vi "VI SysLoad.vi"() -> ()   [LabVIEW 2020, in "Erweiterte Konfig.lvlib" / "System Load.lvlib"]
uses:
  System Load.lvlib
  CPU Status.ctl
  CPU Speicher Auslastung.ctl
  <vilib>/nisyscfg/Close (System).vi
  Allgemein/allgemeine Sub-VIs.lvlib
  <vilib>/nisyscfg/nisyscfg.lvlib
  cRIO/PC/Kommunikation mit cRIO.lvlib
panel:
  out "CPU 2 Load:":T1
  out "Speicher":T2 caption="Memory:"
  out "CPU 1 Load":T1 caption="CPU 1 Load:"
  # "System Load"
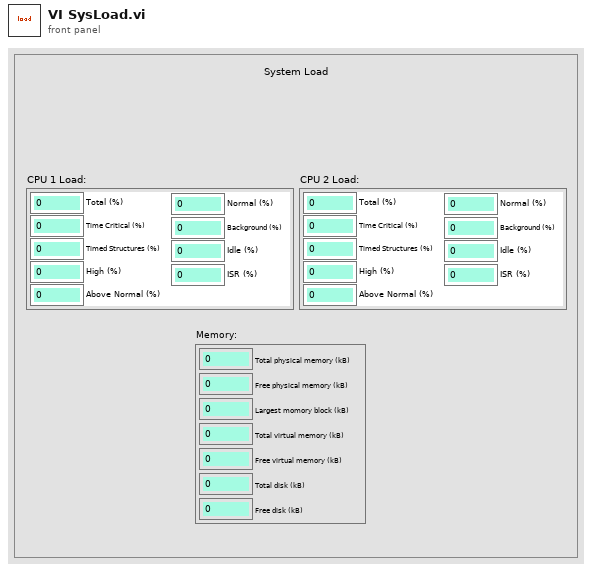
[diagram p1: front panel]
types:
  T1 = typedef "Erweiterte Konfig.lvlib/System Load.lvlib/CPU Status.ctl" = cluster{"Total (%)":sgl, "Time Critical (%)":sgl, "Timed Structures (%)":sgl, "High (%)":sgl, "Above Normal (%)":sgl, "Normal (%)":sgl, "Background (%)":sgl, "Idle (%)":sgl, "ISR (%)":sgl}
  T2 = typedef "Erweiterte Konfig.lvlib/System Load.lvlib/CPU Speicher Auslastung.ctl" = cluster{"Total physical memory (kB)":u32, "Free physical memory (kB)":u32, "Largest momory block (kB)":u32, "Total virtual memory (kB)":u32, "Free virtual memory (kB)":u32, "Total disk (kB)":u32, "Free disk (kB)":u32}
  T3 = cluster{"[0]":sgl, "[1]":sgl, "[2]":sgl, "[3]":sgl, "[4]":sgl, "[5]":sgl, "[6]":sgl, "[7]":sgl, "[8]":sgl}
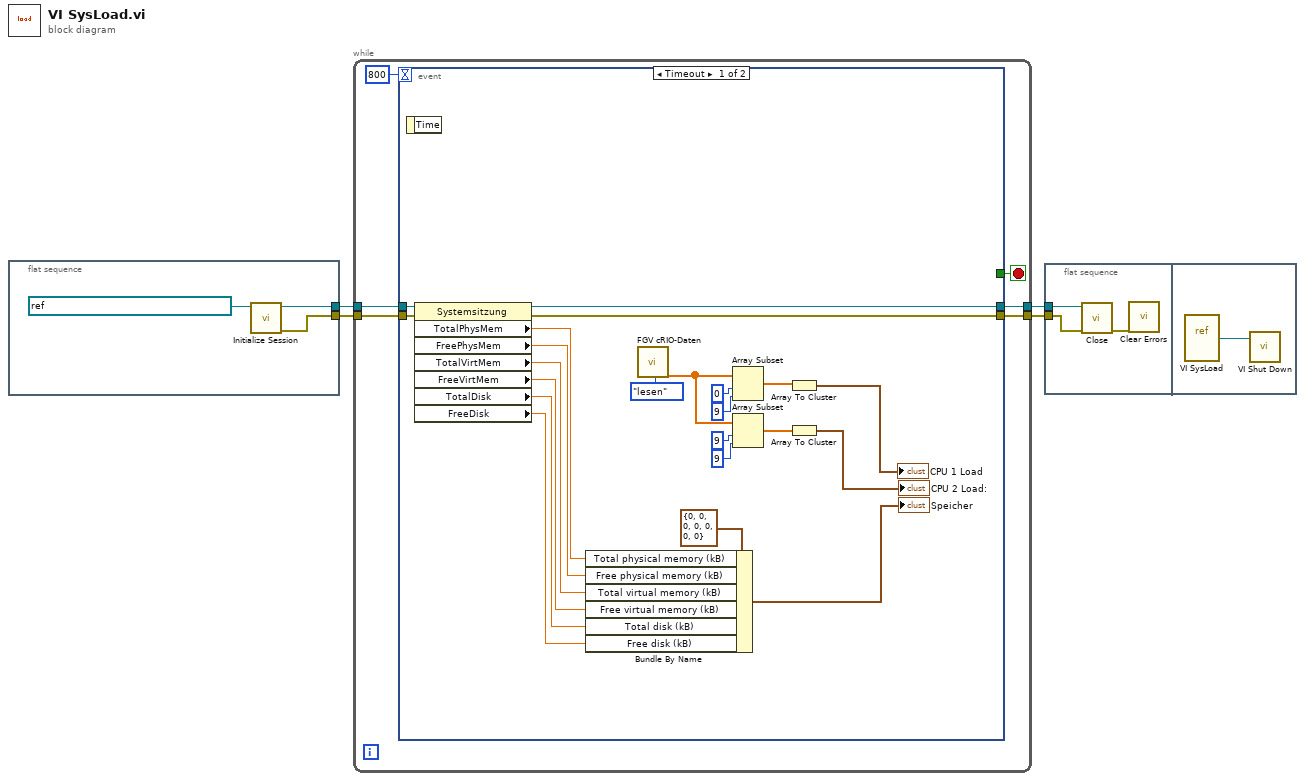
[diagram p0: block diagram]
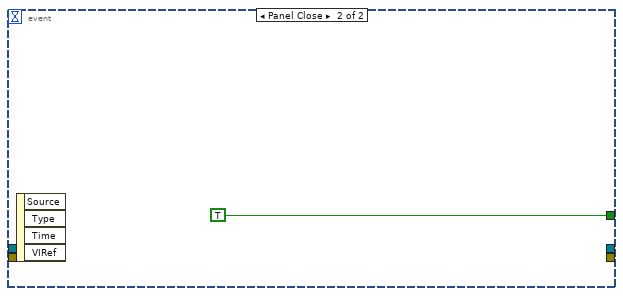
[diagram p2: hidden frame]
diagram:
  n1 = flat-sequence {
    tunnel: [w7] -> w4
    tunnel: [w6] -> w3
    frame #0 {
      n2 = call <vilib>:"Initialize Session.vi"("Target (localhost)"=refnum<k21> "NI-cRIO-9066-IAG (192.168.14.14)") -> ("error out"=w6:errorcluster, "Session out"=w7:refnum<k21>)  [unwired: 9 in]
    }
  }
  n3 = while {
    tunnel: w4 -> [w11]
    tunnel: w3 -> [w10]
    tunnel: [w9] -> w2
    tunnel: [w8] -> w1
    stop <- w12 stop-if-true
    n4 = event shown="[0] Timeout" {
      selector: _ -> [_ _]
      dyn-events: _ -> [_ _]
      timeout: 800 -> [_ _]
      tunnel: [_ TRUE] -> w12
      tunnel: w11 -> [w35 _]
      tunnel: w10 -> [w34 _]
      tunnel: [w33 _] -> w9
      tunnel: [w32 _] -> w8
      event Timeout {
        n5 = event-data() -> ()  [unwired: 1 in, 1 out]
        n6 = property class="Systemsitzung"(reference=w35, error in=w34) -> (reference out=w33:refnum<k21>, error out=w32:errorcluster, "TotalPhysMem"=w31:dbl, "FreePhysMem"=w30:dbl, "TotalVirtMem"=w29:dbl, "FreeVirtMem"=w28:dbl, "TotalDisk"=w27:dbl, "FreeDisk"=w26:dbl)
        n7 = Bundle By Name(cluster=T2 {"Total physical memory (kB)"=0, "Free physical memory (kB)"=0, "Largest momory block (kB)"=0, "Total virtual memory (kB)"=0, "Free virtual memory (kB)"=0, "Total disk (kB)"=0, "Free disk (kB)"=0} ("Speicher"), "Total physical memory (kB)"=w31, "Free physical memory (kB)"=w30, "Total virtual memory (kB)"=w29, "Free virtual memory (kB)"=w28, "Total disk (kB)"=w27, "Free disk (kB)"=w26) -> (→"Speicher":T2)
        n8 = call "FGV cRIO-Daten.vi"("Aktion"=enum16{"lesen", "schreiben"}."lesen") -> ("CPU Status"=w16:sgl[])  [unwired: 9 in, 9 out]
        n9 = Array Subset(array=w16, index=0 ("Index"), length=9 ("Länge")) -> (w20:sgl[])
        n10 = Array Subset(array=w16, index=9 ("Index"), length=9 ("Länge")) -> (w17:sgl[])
        n11 = Array To Cluster(array=w20) -> (cluster=→"CPU 1 Load":T3)
        n12 = Array To Cluster(array=w17) -> (cluster=→"CPU 2 Load:":T3)
      }
      event Panel Close {
        n13 = event-data() -> ()  [unwired: 1 in, 4 out]
      }
    }
  }
  n14 = flat-sequence {
    tunnel: w2 -> [w39]
    tunnel: w1 -> [w38]
    frame #0 {
      n15 = call-poly <vilib>:"Close.vi"("error in (no error)"=w38, "Session in"=w39) -> ("error out"=w37:errorcluster)  [unwired: 9 in]
      n16 = call <vilib>:"Clear Errors.vi"("error in (no error)"=w37) -> ()  [unwired: 5 in, 2 out]
    }
    frame #1 {
      n17 = vi-ref "VI SysLoad.vi"() -> (w40:refnum<vi>)
      n18 = call "VI Shut Down.vi"("VI Referenz"=w40) -> ()  [unwired: 11 in]
    }
  }
